vi "GTH_V2.Record2CalibrationPara.vi"(7 "Calibration Date":bool=TRUE, 8 "错误输入":errorcluster, 9 "Calibration Cycle(Days)":u32=365 min=365 step=1, 10 "Calibration Info":string[](array[string]), 11 "CMD":T1(ring)) -> (0 "错误输出":errorcluster, 2 "Para":dbl[](array[numeric]), 3 "OK?":bool)   [LabVIEW 2012, in "Lib_UEL.ATE.lvlib" / "STM32-CoreBD.lvlib"]
uses:
  STM32-CoreBD.lvlib
  <vilib>/Utility/error.llb/whitespace.ctl
  <vilib>/Utility/miscctls.llb/LVDateTimeRec.ctl
panel:
  # "V1.0.0 初始版本. ~LG,2015-08-13\nCalibration Info需要验证的信息:\n- 校验日期\n- 有对应通道\n- 修正参数Para1不为0"
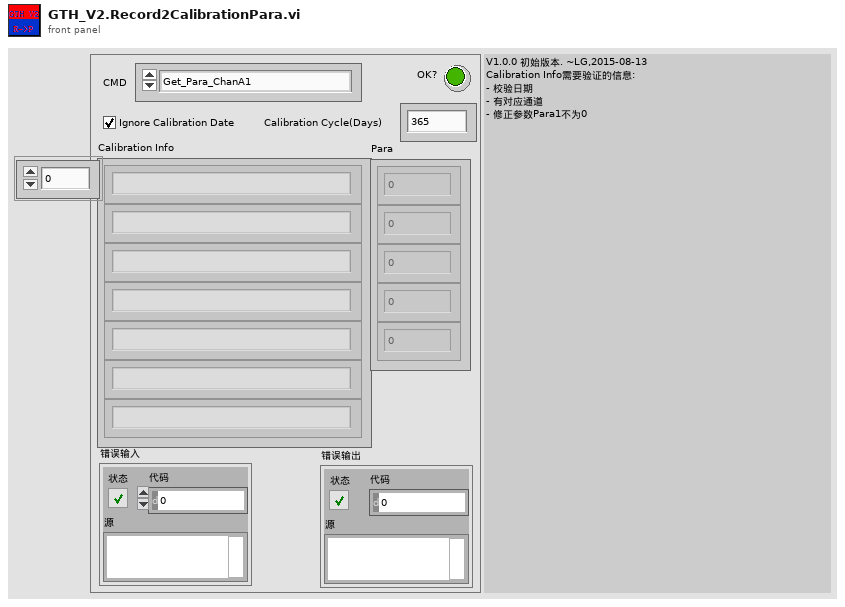
[diagram p1: front panel]
types:
  T1 = enum16{"Get_Para_ChanA1", "Get_Para_ChanA2", "Get_Para_ChanB1", "Get_Para_ChanB2", "Get_Para_ChanC1", "Get_Para_ChanC2", "Get_Para_DAC"}
  T2 = typedef "LVDateTimeRec.ctl" = cluster{"fractional second":dbl, "second":i32, "minute":i32, "hour":i32, "day of month":i32, "month":i32, "year":i32, "day of week":i32, "day of year":i32, "DST":i32}
  T3 = typedef "whitespace.ctl" = u16
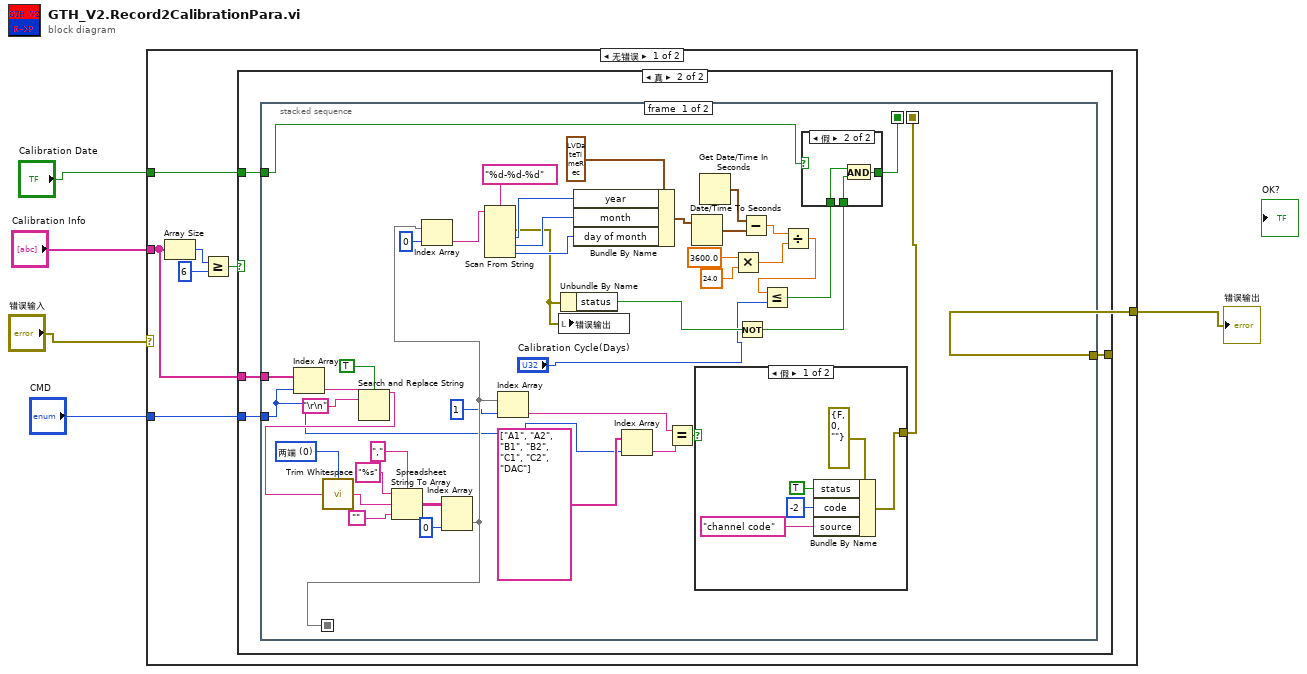
[diagram p0: block diagram]
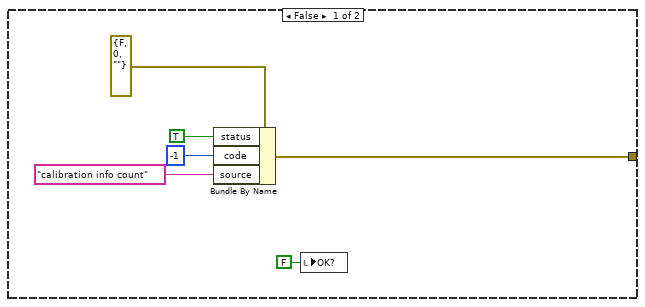
[diagram p2: hidden frame]
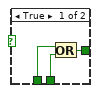
[diagram p3: hidden frame]
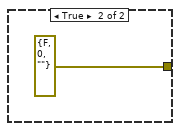
[diagram p4: hidden frame]
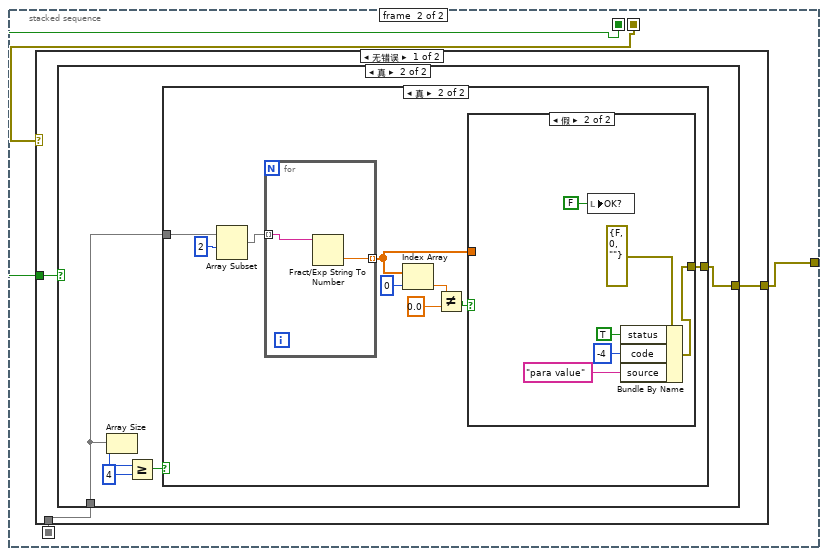
[diagram p5: hidden frame]
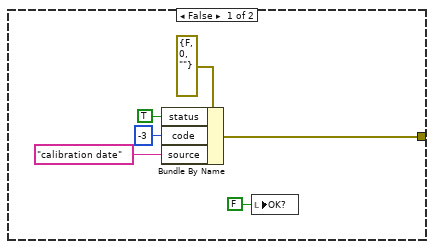
[diagram p6: hidden frame]
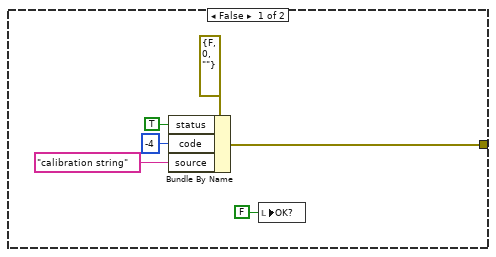
[diagram p7: hidden frame]
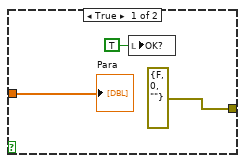
[diagram p8: hidden frame]
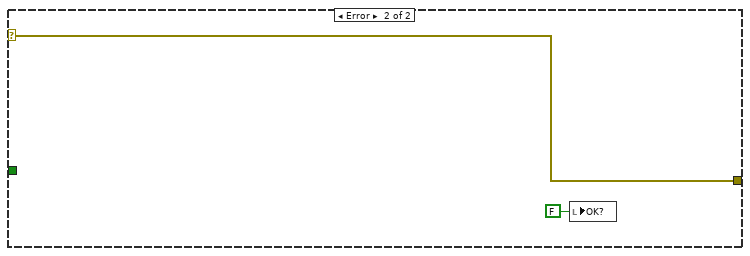
[diagram p9: hidden frame]
diagram:
  n1 = case shown="无错误" "错误输入" {
    selector: "错误输入" -> [_ w123]
    tunnel: [w6 w123] -> w4
    tunnel: "Calibration Info" -> [w12 _]
    tunnel: "Calibration Date" -> [w11 _]
    tunnel: "CMD" -> [w10 _]
    frame No Error {
      n2 = Array Size(array=w12) -> (size(s)=w9:i32)
      n3 = Greater Or Equal?(x=w9, y=6) -> (x >= y?=w7:bool)
      n4 = case shown="真" w7 {
        tunnel: [w17 w19] -> w6
        tunnel: w11 -> [_ w20]
        tunnel: w12 -> [_ w22]
        tunnel: w10 -> [_ w21]
        frame False {
          n5 = Bundle By Name(cluster=errorcluster {"status"=FALSE, "code"=0, "source"=""} ("错误输出"), "status"=TRUE, "code"=-1, "source"="calibration info count") -> (w17:errorcluster)
          n6 = local write "OK?"(FALSE ("OK?")) -> ()
        }
        frame True {
          n7 = stacked-sequence {
            seq-local: [w24 _] -> [_ w80]
            seq-local: [w52 _] -> [_ w78]
            seq-local: [w45 _] -> [_ w77]
            tunnel: w22 -> [w64 _]
            tunnel: w21 -> [w49 _]
            tunnel: w20 -> [w27 _]
            tunnel: [_ w79] -> w19
            frame #0 {
              w59 = T3 0 items=["两端", "字符串首端", "字符串末端"] ("location (both)")
              n8 = Index Array(array=w64, index=w49) -> (element=w63:string)
              n9 = Search and Replace String(case sensitive?=TRUE ("忽略大小写？(F)"), input string=w63, search string="\r\n") -> (result string=w60:string)  [unwired: 5 in, 3 out]
              n10 = call <vilib>:"Trim Whitespace.vi"("string"=w60, "location (both)"=w59) -> ("trimmed string"=w58:string)
              n11 = Spreadsheet String To Array(delimiter (Tab)="," ("分隔符(Tab)"), format string="%s" ("格式字符串"), spreadsheet string=w58, array type (2D Dbl)="") -> (array=w55:string[][])
              n12 = Index Array(array=w55, index (row)=0 ("索引 (行)")) -> (element=w52:string[])  [unwired: 1 in]
              n13 = Index Array(array=w52, index=0 ("索引")) -> (element=w39:string)
              n14 = Scan From String(format string="%d-%d-%d" ("格式字符串"), input string=w39) -> (error out=w29:errorcluster, output 1=w42:i32, output 2=w41:i32, output 3=w40:i32)  [unwired: 5 in, 2 out]
              n15 = Index Array(array=w52, index=1 ("索引")) -> (element=w47:string)
              n16 = local write "错误输出"(w29) -> ()
              n17 = Unbundle By Name(w29) -> ("status"=w28:bool)
              n18 = Bundle By Name(cluster=T2 {"fractional second"=0.0, "second"=0, "minute"=0, "hour"=0, "day of month"=0, "month"=0, "year"=0, "day of week"=0, "day of year"=0, "DST"=0} ("日期时间记录"), "year"=w42, "month"=w41, "day of month"=w40) -> (w37:T2)
              n19 = Index Array(array=string[] ["A1", "A2", "B1", "B2", "C1", "C2", "DAC"], index=w49) -> (element=w48:string)
              n20 = Equal?(x=w47, y=w48) -> (x = y?=w46:bool)
              n21 = Date/Time To Seconds(2:w37) -> (0:w35:timestamp)  [unwired: 1 in]
              n22 = case shown="假" w46 {
                tunnel: [w71 errorcluster {"status"=FALSE, "code"=0, "source"=""} ("错误输出")] -> w45
                frame False {
                  n23 = Bundle By Name(cluster=errorcluster {"status"=FALSE, "code"=0, "source"=""} ("错误输出"), "status"=TRUE, "code"=-2, "source"="channel code") -> (w71:errorcluster)
                }
                frame True {
                }
              }
              n24 = Get Date/Time In Seconds() -> (seconds since 1Jan1904=w36:timestamp)
              n25 = Multiply(x=3600.0, y=24.0 ("x")) -> (x*y=w31:dbl)
              n26 = Not(x=w28) -> (.not. x?=w25:bool)
              n27 = Subtract(x=w36, y=w35) -> (x-y=w32:dbl)
              n28 = Divide(x=w32, y=w31) -> (x/y=w30:dbl)
              n29 = Less Or Equal?(x=w30, y="Calibration Cycle(Days)") -> (x <= y?=w26:bool)
              n30 = case shown="假" w27 {
                tunnel: w26 -> [w67 w70]
                tunnel: w25 -> [w66 w69]
                tunnel: [w65 w68] -> w24
                frame True {
                  n31 = Or(x=w67, y=w66) -> (x .or. y?=w65:bool)
                }
                frame False {
                  n32 = And(x=w70, y=w69) -> (x .and. y?=w68:bool)
                }
              }
            }
            frame #1 {
              n33 = case shown="无错误" w77 {
                selector: w77 -> [_ w122]
                tunnel: w80 -> [w83 _]
                tunnel: [w82 w122] -> w79
                tunnel: w78 -> [w81 _]
                frame No Error {
                  n34 = case shown="真" w83 {
                    tunnel: [w85 w91] -> w82
                    tunnel: w81 -> [_ w90]
                    frame False {
                      n35 = Bundle By Name(cluster=errorcluster {"status"=FALSE, "code"=0, "source"=""} ("错误输出"), "status"=TRUE, "code"=-3, "source"="calibration date") -> (w85:errorcluster)
                      n36 = local write "OK?"(FALSE ("OK?")) -> ()
                    }
                    frame True {
                      n37 = Array Size(array=w90) -> (size(s)=w94:i32)
                      n38 = Greater Or Equal?(x=w94, y=4) -> (x >= y?=w92:bool)
                      n39 = case shown="真" w92 {
                        tunnel: [w95 w106] -> w91
                        tunnel: w90 -> [_ w109]
                        frame False {
                          n40 = Bundle By Name(cluster=errorcluster {"status"=FALSE, "code"=0, "source"=""} ("错误输出"), "status"=TRUE, "code"=-4, "source"="calibration string") -> (w95:errorcluster)
                          n41 = local write "OK?"(FALSE ("OK?")) -> ()
                        }
                        frame True {
                          n42 = Array Subset(array=w109, index=2 ("索引")) -> (w107:string[])  [unwired: 1 in]
                          n43 = for {
                            tunnel: w107 -> [w120] mode=indexing
                            tunnel: [w119] -> w105 mode=indexing
                            n44 = Fract/Exp String To Number(string=w120) -> (number=w119:dbl)  [unwired: 3 in, 1 out]
                          }
                          n45 = Index Array(array=w105, index=0 ("索引")) -> (element=w103:dbl)
                          n46 = Not Equal?(x=w103, y=0.0) -> (x != y?=w101:bool)
                          n47 = case shown="假" w101 {
                            tunnel: [errorcluster {"status"=FALSE, "code"=0, "source"=""} ("错误输出") w113] -> w106
                            tunnel: w105 -> [w110 _]
                            frame True {
                              n48 = local write "OK?"(TRUE ("OK?")) -> ()
                              "Para" <- w110
                            }
                            frame False {
                              n49 = local write "OK?"(FALSE ("OK?")) -> ()
                              n50 = Bundle By Name(cluster=errorcluster {"status"=FALSE, "code"=0, "source"=""} ("错误输出"), "status"=TRUE, "code"=-4, "source"="para value") -> (w113:errorcluster)
                            }
                          }
                        }
                      }
                    }
                  }
                }
                frame Error {
                  n51 = local write "OK?"(FALSE ("OK?")) -> ()
                }
              }
            }
          }
        }
      }
    }
    frame Error {
    }
  }
  "错误输出" <- w4
